vi "Main.vi"() -> ()   [LabVIEW 2018]
panel:
  in  "stop":bool
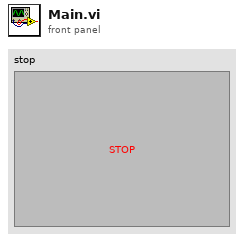
[diagram p1: front panel]
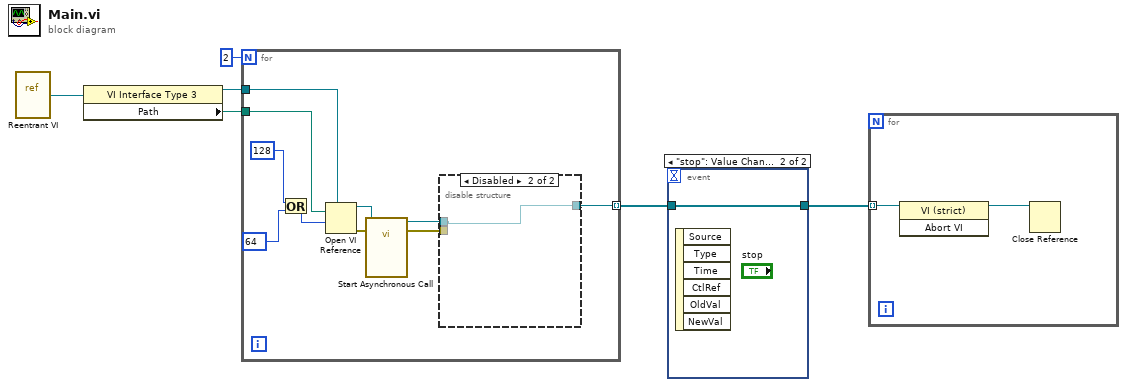
[diagram p0: block diagram]
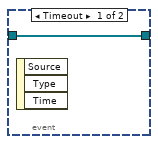
[diagram p2: hidden frame]
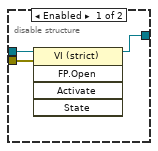
[diagram p3: hidden frame]
diagram:
  n1 = vi-ref "Reentrant VI.vi"() -> (w6:refnum<vi>)
  n2 = property class="VI Interface Type 3"(reference=w6) -> (reference out=w1:refnum<vi>, "Path"=w5:path)  [unwired: 1 in, 1 out]
  n3 = for {
    N: 2 -> [_]
    tunnel: w5 -> [w16]
    tunnel: [w8] -> w3 mode=indexing
    tunnel: w1 -> [w15]
    n4 = Or(x=128, y=64 ("options")) -> (x .or. y?=w12:i32)
    n5 = Open VI Reference(type specifier VI Refnum (for type only)=w15, vi path=w16, options=w12) -> (vi reference=w11:refnum<vi>, error out=w10:errorcluster)  [unwired: 3 in]
    n6 = call-by-ref "Start Asynchronous Call"(reference=w11, error in=w10) -> (reference out=w9:refnum<vi>, error out=w7:errorcluster)  [unwired: 12 in]
    n7 = disable-structure shown="Disabled" {
      disable-tunnel: w9 -> [w19 w20]
      disable-tunnel: [w18 w20] -> w8
      disable-tunnel: w7 -> [w17 _]
      frame Enabled {
        n8 = invoke class="VI (strict)" method="FP.Open"(reference=w19, error in=w17) -> (reference out=w18:refnum<vi>)  [unwired: 3 in, 4 out]
      }
      frame Disabled {
      }
    }
  }
  n9 = event shown="[1] \"stop\": Value Change" {
    selector: _ -> [_ _]
    dyn-events: _ -> [_ _]
    timeout: _ -> [_ _]
    tunnel: [w21 w22] -> w2
    tunnel: w3 -> [w21 w22]
    event Timeout {
      n10 = event-data() -> ()  [unwired: 1 in, 3 out]
    }
    event "stop": Value Change {
      n11 = event-data() -> ()  [unwired: 1 in, 6 out]
    }
  }
  n12 = for {
    tunnel: w2 -> [w23] mode=indexing
    n13 = invoke class="VI (strict)" method="Abort VI"(reference=w23) -> (reference out=w24:refnum<vi>)  [unwired: 2 in, 2 out]
    n14 = Close Reference(reference=w24) -> ()  [unwired: 1 in, 1 out]
  }
